vi "output_conveyor.vi"(11 "Conveyor_outputs":T1) -> (0 "error out":errorcluster)   [LabVIEW 2012]
uses:
  Conveyor_outputs.ctl
  Conveyor module state.ctl
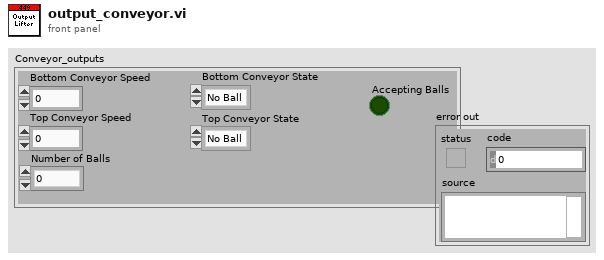
[diagram p1: front panel]
types:
  T1 = typedef "Conveyor_outputs.ctl" = cluster{"Bottom Conveyor Speed":dbl, "Top Conveyor Speed":dbl, "Bottom Conveyor State":T2, "Top Conveyor State":T2, "Accepting Balls":bool, "Number of Balls":i32}
  T2 = typedef "Conveyor module state.ctl" = enum16{"No Ball", "Has Ball", "Ball Below Hold", "Ball Above Hold", "Outputting Ball", "Reset"}
  T3 = typedef "WPI_MotorControlDeviceRef.ctl" = cluster{"DeviceStatus":errorcluster, "Type":enum16{"PWM", "CAN"}, "PWM":cluster{"Digital Module":T4, "PWM Channel":T5, "DeadBand":T6}, "CAN":cluster{"Device Number":u8, "Control Mode":T7, "Semaphore":T8, "Max Vout":dbl}, "Invert":bool, "TransformRef":T9, "InvTransformRef":T9}
  T4 = typedef "FPGA_TypedefDigitalModule.ctl" = enum16{"Digital Module 1", "Digital Module 2"}
  T5 = typedef "FPGA_DIOPWMChannel.ctl" = enum8{"PWM 1", "PWM 2", "PWM 3", "PWM 4", "PWM 5", "PWM 6", "PWM 7", "PWM 8", "PWM 9", "PWM 10", "Invalid"}
  T6 = typedef "WPI_PWMDeadband.ctl" = cluster{"Name":string, "maxPositivePwm":i32, "minPositivePwm":i32, "centerPwm":i32, "maxNegativePwm":i32, "minNegativePwm":i32, "angularRange":u16}
  T7 = typedef "WPI_CANJaguar_ControlMode.ctl" = enum8{"Percent VBus", "Current", "Speed", "Position", "Voltage"}
  T8 = typedef "Semaphore RefNum" = refnum<k1>
  T9 = typedef "WPI_PWMTransform_ConPane.ctl" = refnum<vi>
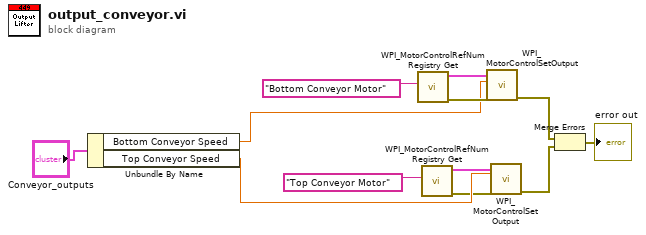
[diagram p0: block diagram]
diagram:
  n1 = Unbundle By Name("Conveyor_outputs") -> ("Bottom Conveyor Speed"=w6:dbl, "Top Conveyor Speed"=w5:dbl)
  n2 = call <vilib>:"WPI_MotorControlRefNum Registry Get.vi"("refnum name"="Bottom Conveyor Motor") -> ("error out"=w9:errorcluster, "MotorControlDevRef"=w12:T3)  [unwired: 9 in]
  n3 = call <vilib>:"WPI_MotorControlRefNum Registry Get.vi"("refnum name"="Top Conveyor Motor") -> ("error out"=w1:errorcluster, "MotorControlDevRef"=w3:T3)  [unwired: 9 in]
  n4 = call <vilib>:"WPI_MotorControlSetOutput.vi"("error in (no error)"=w9, "Output"=w6, "MotorControlDevRef"=w12) -> ("error out"=w8:errorcluster)  [unwired: 6 in, 2 out]
  n5 = call <vilib>:"WPI_MotorControlSetOutput.vi"("error in (no error)"=w1, "Output"=w5, "MotorControlDevRef"=w3) -> ("error out"=w4:errorcluster)  [unwired: 6 in, 2 out]
  n6 = Merge Errors(w8, w4) -> (→"error out":errorcluster)
